vi "Cheby Pade fit.vi"(0 "start":dbl=70.0 format="%.2f", 1 "order":u32=6, 2 "number of points":u32=56, 5 "end":dbl=150.0 format="%.2f", 7 "X-array":dbl[](array[numeric]), 9 "Y-array":dbl[](array[numeric]), 12 "p-the derivative":i32=10, 13 "m":i32=5, 14 "n":i32=5) -> (4 "Tn coeffs":dbl[](array[numeric])=[31.19495843473104, -3.275952846439739, 0.1987322533001959, 0.06629653556908306, -0.054416194384996786, 0.010595544376378996] format="%.2f", 6 "Numerator":dbl[](array[numeric])=[15.597479217365517, -3.4218647312650936, 0.8327940616803662, 0.053275254748753026, -0.43532955507997295, 0.16952871002206407] format="%.6f", 8 "Denominator":dbl[](array[numeric])=[1.0, 0.0, 0.0, 0.0, 0.0, 0.0] format="%.6f", 10 "XY Graph":cluster{dbl[], dbl[]}[](graph)=[{[0.47166, 0.48675, 0.50232, 0.5184, 0.53498, 0.5521, 0.56976, 0.588, 0.60681, 0.62622, 0.64626, 0.66694, 0.68828, 0.7103, 0.73303, 0.75648, 0.78068, 0.80566, 0.83144, 0.85804, 0.8855, 0.91383, 0.94307, 0.97325, 1.00439, 1.03652, 1.06969, 1.10391, 1.13923, 1.17568, 1.2133, 1.25212, 1.29219, 1.33353, 1.3762, 1.42023, 1.46567, 1.51257, 1.56097, 1.61091, 1.66245, 1.71565, 1.77054, 1.82719, 1.88565, 1.94599, 2.00825, 2.07251, 2.13882, 2.20725, 2.27788, 2.35076, 2.42598, 2.5036, 2.5837, 2.66637, 2.75169, 2.83973, 2.93059, 3.02436, 3.12113, 3.22099, 3.32405, 3.43041, 3.54017, 3.65344, 3.77033, 3.89097, 4.01547, 4.14395, 4.27654, 4.41337, 4.55458, 4.70031, 4.8507, 5.0059, 5.16607, 5.33137, 5.50195, 5.67799, 5.85967, 6.04715, 6.24064, 6.44032, 6.64638, 6.85904, 7.0785, 7.30499, 7.53872, 7.77993, 8.02886, 8.28575, 8.55086, 8.82445, 9.1068, 9.39819, 9.69889, 10.0092, 10.3295, 10.66, 11.0011, 11.353, 11.7163, 12.0912, 12.4781, 12.8773, 13.2893, 13.7145, 14.1533, 14.6062, 15.0735, 15.5558, 16.0536, 16.5672, 17.0973, 17.6443, 18.2089, 18.7915, 19.3928, 20.0133, 20.6536, 21.3144, 21.9964, 22.7002, 23.4265, 24.1761, 24.9496, 25.7479, 26.5718, 27.422, 28.2994, 29.2048, 30.1393, 31.1036, 32.0988, 33.1259, 34.1858, 35.2796, 36.4084, 37.5733, 38.7755, 40.0162, 41.2965, 42.6179, 43.9815, 45.3887, 46.841, 48.3397, 49.8864, 51.4826, 53.1298, 54.8298, 56.5841, 58.3946, 60.263, 62.1912, 64.181, 66.2346, 68.3538, 70.5409, 72.7979, 75.1272, 77.531, 80.0117, 82.5717, 85.2137, 87.9402, 90.754, 93.6577, 96.6544, 99.747, 102.939, 106.232, 109.631, 113.139, 116.759, 120.495, 124.35, 128.329, 132.435, 136.672, 141.045, 145.558, 150.216, 155.022, 159.982, 165.101, 170.383, 175.835, 181.461, 187.267, 193.259, 199.442, 205.824, 212.409, 219.206, 226.219, 233.458, 240.927, 248.636], [0.04369, 0.04561, 0.0476, 0.04965, 0.05177, 0.05396, 0.05621, 0.0589, 0.06196, 0.06512, 0.06837, 0.07174, 0.07518, 0.07865, 0.08223, 0.08593, 0.08975, 0.09466, 0.10012, 0.10576, 0.11158, 0.11759, 0.12379, 0.13101, 0.13851, 0.14625, 0.15425, 0.16251, 0.17103, 0.18593, 0.20556, 0.22582, 0.24675, 0.26835, 0.29198, 0.31887, 0.34662, 0.37527, 0.40486, 0.4354, 0.46693, 0.50366, 0.5425, 0.5826, 0.62401, 0.66675, 0.70939, 0.75065, 0.79326, 0.83725, 0.88267, 0.92957, 0.98463, 1.05538, 1.12843, 1.20384, 1.28171, 1.3621, 1.44636, 1.53862, 1.63388, 1.73223, 1.83377, 1.93861, 2.04685, 2.1586, 2.27398, 2.3931, 2.53674, 2.69895, 2.86642, 3.03932, 3.21431, 3.39354, 3.57859, 3.76964, 3.96689, 4.13732, 4.29297, 4.45366, 4.61958, 4.79936, 5.00776, 5.22292, 5.44506, 5.63666, 5.7907, 5.94975, 6.119, 6.35913, 6.60705, 6.86211, 6.95953, 7.06011, 7.16396, 7.27118, 7.38188, 7.44894, 7.49568, 7.54569, 7.60164, 7.65941, 7.71342, 7.64668, 7.57777, 7.50663, 7.43318, 7.36236, 7.30161, 7.23888, 7.17412, 7.10726, 7.04646, 6.99619, 6.94428, 6.8907, 6.83537, 6.80319, 6.79324, 6.78296, 6.77236, 6.7614, 6.8054, 6.91834, 7.03494, 7.15532, 7.27962, 7.45801, 7.889, 8.33397, 8.79339, 9.26772, 9.7666, 10.2936, 10.8378, 11.3996, 11.9797, 12.5228, 13.0316, 13.557, 14.0994, 14.6594, 15.2376, 15.7758, 16.1744, 16.5858, 17.0106, 17.4492, 17.765, 18.0492, 18.3427, 18.6457, 18.949, 18.9931, 19.0387, 19.0858, 19.1344, 19.1845, 19.0548, 18.9111, 18.7628, 18.6097, 18.4162, 18.183, 17.9422, 17.6936, 17.4369, 17.1637, 16.8762, 16.5793, 16.2728, 15.9563, 15.6484, 15.3755, 15.0936, 14.8027, 14.5022, 14.1959, 13.9348, 13.6653, 13.387, 13.0997, 12.8156, 12.5313, 12.2378, 11.9348, 11.6219, 11.4173, 11.3293, 11.2384, 11.1446, 11.0478, 10.9478, 10.9239, 10.9096, 10.8949, 10.8797, 10.8641, 11.0173, 11.1932]}, {[70.0, 71.42857142857143, 72.85714285714286, 74.28571428571429, 75.71428571428571, 77.14285714285714, 78.57142857142857, 80.0, 81.42857142857143, 82.85714285714286, 84.28571428571429, 85.71428571428572, 87.14285714285714, 88.57142857142857, 90.0, 91.42857142857143, 92.85714285714286, 94.28571428571428, 95.71428571428572, 97.14285714285714, 98.57142857142857, 100.0, 101.42857142857143, 102.85714285714286, 104.28571428571428, 105.71428571428572, 107.14285714285714, 108.57142857142857, 110.0, 111.42857142857143, 112.85714285714286, 114.28571428571428, 115.71428571428572, 117.14285714285714, 118.57142857142857, 120.0, 121.42857142857143, 122.85714285714286, 124.28571428571428, 125.71428571428572, 127.14285714285714, 128.57142857142856, 130.0, 131.42857142857144, 132.85714285714286, 134.28571428571428, 135.71428571428572, 137.14285714285714, 138.57142857142856, 140.0, 141.42857142857144, 142.85714285714286, 144.28571428571428, 145.71428571428572, 147.14285714285714, 148.57142857142856], [18.940856042774996, 18.8528535998892, 18.756504933447665, 18.65269024488724, 18.542242004472744, 18.425946133342833, 18.30454318555592, 18.17872953013614, 18.04915853311917, 17.916441739598252, 17.781150055770034, 17.643814930980533, 17.50492953977099, 17.364949963923866, 17.224296374508686, 17.083354213927997, 16.942475377963273, 16.80197939782083, 16.662154622177724, 16.523259399227705, 16.38552325872711, 16.24914809404076, 16.11430934418792, 15.98115717588817, 15.849817665607354, 15.720393981603484, 15.592967565972643, 15.467599316694923, 15.344330769680326, 15.223185280814686, 15.10416920800558, 14.987273093228248, 14.872472844571504, 14.759730918283664, 14.648997500818439, 14.540211690880877, 14.433302681473254, 14.328190941941015, 14.224789400018668, 14.123004623875705, 14.022738004162532, 13.923886936056366, 13.826346001307154, 13.730008150283508, 13.634765884018591, 13.540512436256062, 13.447142955495952, 13.354555687040639, 13.262653155040706, 13.171343344540883, 13.08054088352597, 12.99016822496674, 12.900156828865848, 12.810448344303769, 12.720995791484693, 12.631764743782458]}, {[70.0, 71.42857142857143, 72.85714285714286, 74.28571428571429, 75.71428571428571, 77.14285714285714, 78.57142857142857, 80.0, 81.42857142857143, 82.85714285714286, 84.28571428571429, 85.71428571428572, 87.14285714285714, 88.57142857142857, 90.0, 91.42857142857143, 92.85714285714286, 94.28571428571428, 95.71428571428572, 97.14285714285714, 98.57142857142857, 100.0, 101.42857142857143, 102.85714285714286, 104.28571428571428, 105.71428571428572, 107.14285714285714, 108.57142857142857, 110.0, 111.42857142857143, 112.85714285714286, 114.28571428571428, 115.71428571428572, 117.14285714285714, 118.57142857142857, 120.0, 121.42857142857143, 122.85714285714286, 124.28571428571428, 125.71428571428572, 127.14285714285714, 128.57142857142856, 130.0, 131.42857142857144, 132.85714285714286, 134.28571428571428, 135.71428571428572, 137.14285714285714, 138.57142857142856, 140.0, 141.42857142857144, 142.85714285714286, 144.28571428571428, 145.71428571428572, 147.14285714285714, 148.57142857142856], [19.194004490460184, 19.106002047574396, 19.009653381132853, 18.905838692572434, 18.79539045215794, 18.67909458102803, 18.557691633241117, 18.431877977821326, 18.302306980804364, 18.169590187283447, 18.034298503455233, 17.896963378665724, 17.758077987456183, 17.618098411609054, 17.477444822193874, 17.33650266161319, 17.19562382564846, 17.055127845506014, 16.915303069862915, 16.7764078469129, 16.6386717064123, 16.50229654172595, 16.36745779187311, 16.234305623573363, 16.102966113292545, 15.973542429288672, 15.846116013657834, 15.720747764380116, 15.597479217365517, 15.476333728499876, 15.357317655690771, 15.24042154091344, 15.125621292256696, 15.012879365968855, 14.90214594850363, 14.793360138566067, 14.686451129158446, 14.581339389626205, 14.477937847703858, 14.376153071560898, 14.275886451847724, 14.177035383741558, 14.07949444899235, 13.9831565979687, 13.887914331703785, 13.79366088394125, 13.700291403181144, 13.60770413472583, 13.515801602725897, 13.424491792226075, 13.333689331211161, 13.24331667265193, 13.15330527655104, 13.063596791988962, 12.974144239169886, 12.88491319146765]}])   [LabVIEW 2024]
uses:
  Cheby 2D array prep_XY arrays.vi
panel:
  # "1. Note that the Chebyshev approximation is performed for normlaized x, i.e. [-1,1]. \nTherefore, x input for the Pade approximation  also requires the same normalization.\n2. Should be an ascending order"
  # "p=m+n\nm>=n"
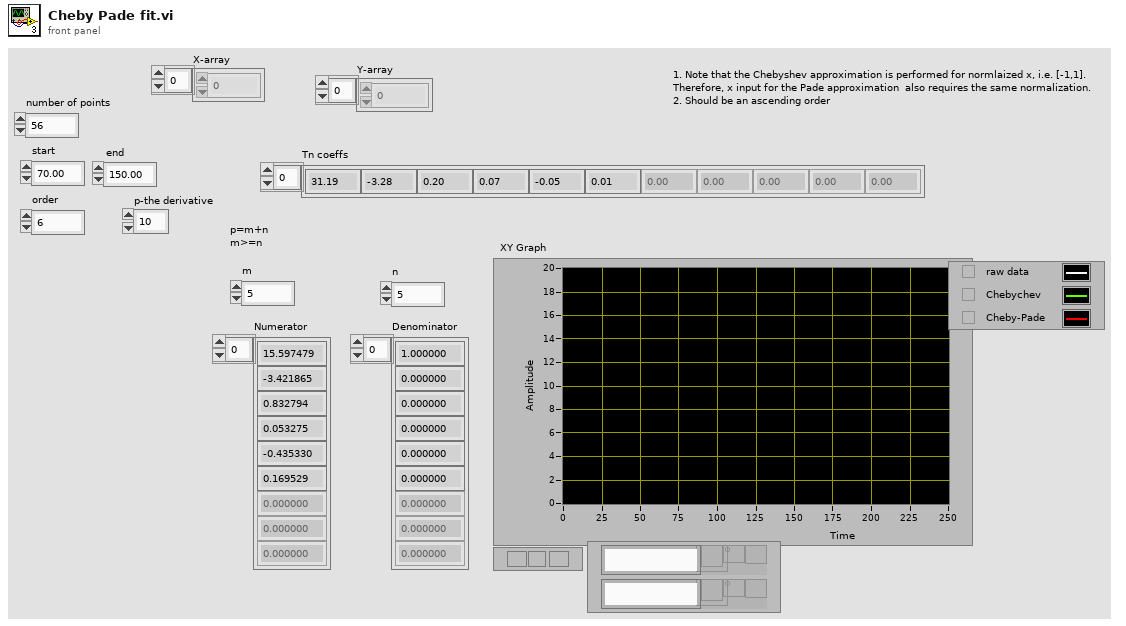
[diagram p1: front panel]
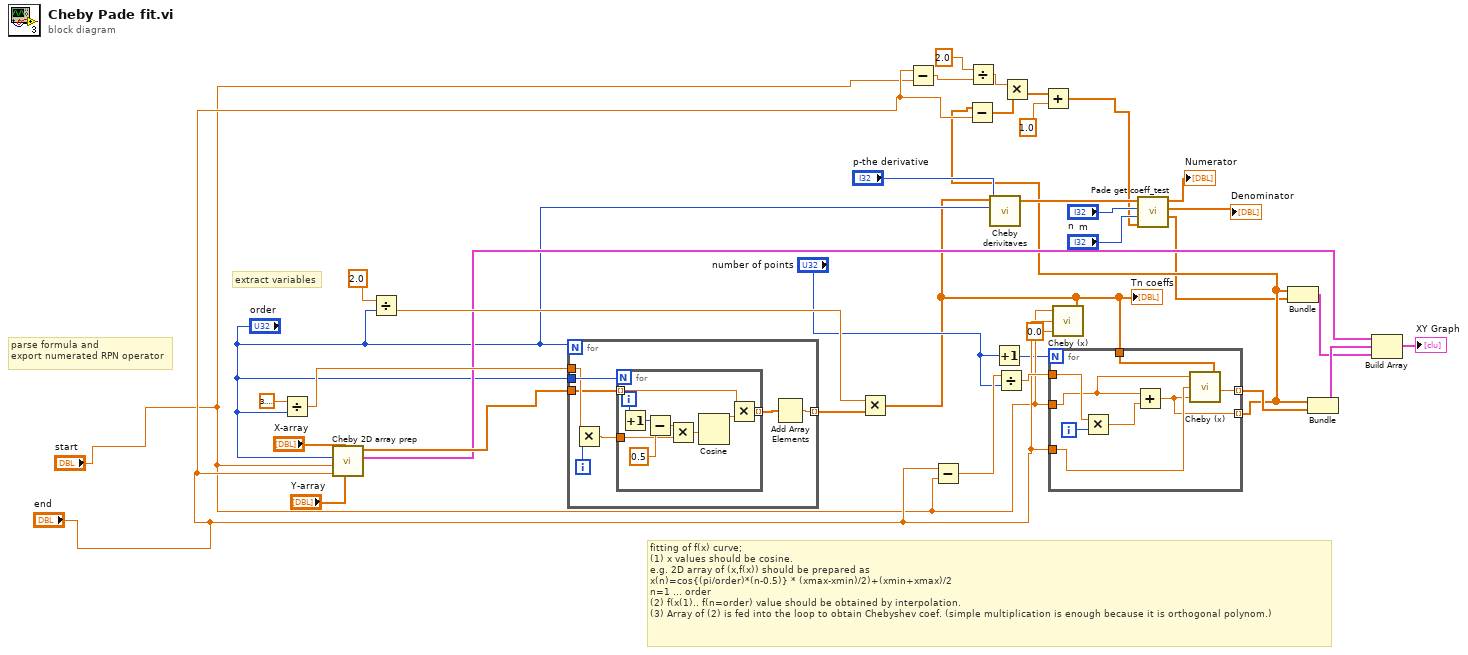
[diagram p0: block diagram]
diagram:
  # "extract variables"
  # "fitting of f(x) curve;\n(1) x values should be cosine.\ne.g. 2D array of (x,f(x)) should be prepared as \nx(n)=cos{(pi/order)*(n-0.5)} * (xmax-xmin)/2)+(xmin+xmax)/2 \nn=1 ... order\n(2) f(x(1).. f(n=order) value should be obtained by interpolation.\n(3) Array of (2) is fed into the loop to obtain Chebyshev coef. (simple multiplication is enough because it is orthogonal polynom.)"
  # "parse formula and\nexport numerated RPN operator"
  n1 = Divide(x=3.141592653589793, y="order") -> (x/y=w33:dbl)
  n2 = call-poly "Cheby 2D array prep.vi"("Y-array"="Y-array", "X-array"="X-array", "end"="end", "start"="start", "order"="order") -> ("original curve"=w30:cluster{dbl[], dbl[]}, "values"=w31:dbl[])  [unwired: 4 in]
  n3 = Divide(x=2.0, y="order") -> (x/y=w35:dbl)
  n4 = for {
    N: "order" -> [_]
    tunnel: "order" -> [w44]
    tunnel: w33 -> [w43]
    tunnel: w31 -> [w41]
    tunnel: [w39] -> w36 mode=indexing
    i -> [w38]
    n5 = Multiply(x=w43, y=w38) -> (x*y=w42:dbl)
    n6 = for {
      N: w44 -> [_]
      tunnel: w42 -> [w45]
      tunnel: w41 -> [w52] mode=indexing
      tunnel: [w51] -> w40 mode=indexing
      i -> [w50]
      n7 = Increment(x=w50) -> (x+1=w46:i32)
      n8 = Subtract(x=w46, y=0.5) -> (x-y=w48:dbl)
      n9 = Multiply(x=w48, y=w45) -> (x*y=w47:dbl)
      n10 = Cosine(x=w47) -> (cos(x)=w53:dbl)
      n11 = Multiply(x=w52, y=w53) -> (x*y=w51:dbl)
    }
    n12 = Add Array Elements(numeric array=w40) -> (sum=w39:dbl)
  }
  n13 = Multiply(x=w35, y=w36) -> (x*y=w9:dbl[])
  "Tn coeffs" <- w9
  n14 = Subtract(x="end", y="start") -> (x-y=w19:dbl)
  n15 = Subtract(x="end", y="start") -> (x-y=w29:dbl)
  n16 = Divide(x=2.0, y=w19) -> (x/y=w17:dbl)
  n17 = call "Cheby derivitaves.vi"("p-the derivative"="p-the derivative", "Cheby order n"="order", "Coeff"=w9) -> ("Derivatives"=w24:dbl[])  [unwired: 8 in]
  n18 = Increment(x="number of points") -> (x+1=w1:u32)
  n19 = Divide(x=w29, y="number of points") -> (x/y=w27:dbl)
  n20 = for {
    N: w1 -> [_]
    tunnel: "start" -> [w58]
    tunnel: w27 -> [w61]
    tunnel: "end" -> [w57]
    tunnel: w9 -> [w56]
    tunnel: [w55] -> w26 mode=indexing
    tunnel: [w54] -> w3 mode=indexing
    i -> [w60]
    n21 = Multiply(x=w61, y=w60) -> (x*y=w59:dbl)
    n22 = Add(x=w58, y=w59) -> (x+y=w54:dbl)
    n23 = call "Cheby (x).vi"("Tn coeffs"=w56, "x"=w54, "end"=w57, "start"=w58) -> ("f(x)"=w55:dbl)
  }
  n24 = Subtract(x=w3, y="end") -> (x-y=w16:dbl[])
  n25 = Multiply(x=w17, y=w16) -> (x*y=w15:dbl[])
  n26 = Add(x=w15, y=1.0) -> (x+y=w13:dbl[])
  n27 = call "Cheby (x).vi"("Tn coeffs"=w9, "x"=0.0, "end"="end", "start"="start") -> ()  [unwired: 1 out]
  n28 = call "Pade get coeff_test.vi"("x array"=w13, "n"="n", "m"="m", "Derivatives"=w24) -> ("Pade_mn array"=w2:dbl[], "Denominator"=→"Denominator":dbl[], "Numerator"=→"Numerator":dbl[])  [unwired: 4 in, 1 out]
  n29 = Bundle(w3, "Pade_mn array"=w2) -> (w12:cluster{dbl[], "Pade_mn array":dbl[]})  [unwired: 1 in]
  n30 = Bundle(w3, w26) -> (w25:cluster{dbl[], dbl[]})  [unwired: 1 in]
  n31 = Build Array(w30, w25, w12) -> (→"XY Graph":cluster{dbl[], "Pade_mn array":dbl[]}[])
